vi "Set Scaling (MapRange).vi"(7 "Scaled Units":string, 8 "error in (no error)":errorcluster, 9 "Range":T1={"Minimum"=-5.0, "Maximum"=5.0}, 10 "Scale Name":string, 11 "DAQmx-AI":refnum<class "DAQmx-AI.lvclass">) -> (0 "error out":errorcluster, 3 "DAQmx-AI out":refnum<class "DAQmx-AI.lvclass">)   [LabVIEW 2016, in "DAQmx-AI.lvclass"]
uses:
  DAQmx-AI.lvclass
  Typedefs/Scaling(MapRange)--Cluster.ctl
  Typedefs/ScalingType--Enum.ctl
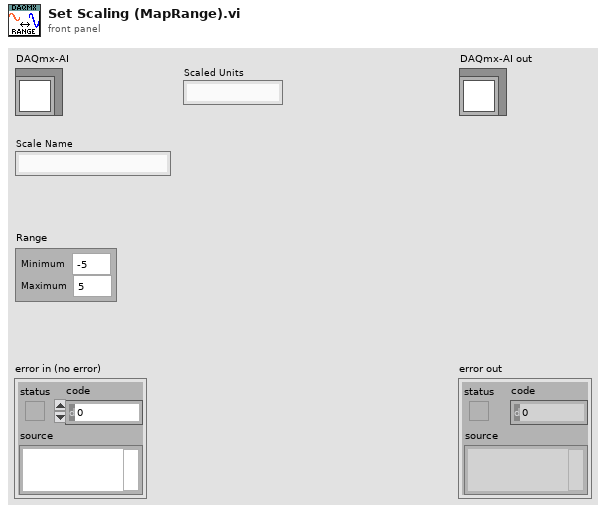
[diagram p1: front panel]
types:
  T1 = typedef "DAQmx-AI.lvclass/Scaling(MapRange)--Cluster.ctl" = cluster{"Minimum":dbl, "Maximum":dbl}
  T2 = typedef "DAQmx-AI.lvclass/ScalingType--Enum.ctl" = enum16{"No scaling", "Linear", "Map Range", "Polynomial", "Table"}
  T3 = typedef "DAQmx-AI.lvclass/Scaling--Cluster.ctl" = cluster{"Scale Name":string, "Scale Type":T2, "Scaled Units":string, "Linear":T4, "Map Range":T1, "Polynomial":T5, "Table":T6}
  T4 = typedef "DAQmx-AI.lvclass/Scaling(Linear)--Cluster.ctl" = cluster{"Slope":dbl, "Intercept":dbl}
  T5 = typedef "DAQmx-AI.lvclass/Scaling(Polynomial)--Cluster.ctl" = cluster{"forward coeff":dbl[], "reverse coeff":dbl[]}
  T6 = typedef "DAQmx-AI.lvclass/Scaling(Table)--Cluster.ctl" = cluster{"scaled values":dbl[], "pres-scaled values":dbl[]}
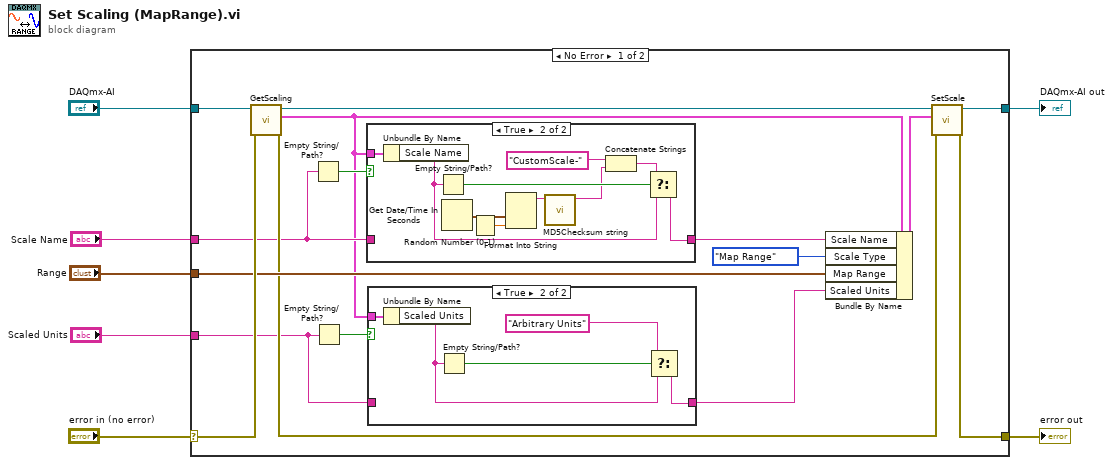
[diagram p0: block diagram]
diagram:
  n1 = case shown="No Error" "error in (no error)" {
    selector: "error in (no error)" -> [w19 w42]
    tunnel: [w22 w42] -> w6
    tunnel: [w23 w41] -> w4
    tunnel: "DAQmx-AI" -> [w21 w41]
    tunnel: "Scale Name" -> [w13 _]
    tunnel: "Scaled Units" -> [w8 _]
    tunnel: "Range" -> [w17 _]
    frame No Error {
      n2 = call "GetScaling.vi"("error in (no error)"=w19, "DAQmx-AI"=w21) -> ("error out"=w15:errorcluster, "Scaling"=w10:T3, "DAQmx-AI out"=w20:refnum<class "DAQmx-AI.lvclass">)  [unwired: 6 in, 1 out]
      n3 = Empty String/Path?(string/path=w13) -> (empty?=w14:bool)
      n4 = Empty String/Path?(string/path=w8) -> (empty?=w11:bool)
      n5 = case shown="True" w14 {
        tunnel: w10 -> [_ w40]
        tunnel: w13 -> [w30 _]
        tunnel: [w30 w37] -> w12
        frame False {
        }
        frame True {
          n6 = Unbundle By Name(w40) -> ("Scale Name"=w38:string)
          n7 = Empty String/Path?(string/path=w38) -> (empty?=w39:bool)
          n8 = Get Date/Time In Seconds() -> (seconds since 1Jan1904=w36:timestamp)
          n9 = Random Number (0-1)() -> (number: 0 to 1=w35:dbl)
          n10 = Format Into String(w36, w35) -> (resulting string=w34:string)  [unwired: 3 in, 1 out]
          n11 = call <vilib>:"MD5Checksum string.vi"("Message String"=w34) -> ("MD5 message-digest"=w32:string)  [unwired: 10 in]
          n12 = Concatenate Strings("CustomScale-" ("t"), w32) -> (w31:string)
          n13 = Select(t=w31, s=w39, f=w38) -> (s? t:f=w37:string)
        }
      }
      n14 = case shown="True" w11 {
        tunnel: w10 -> [_ w29]
        tunnel: w8 -> [w24 _]
        tunnel: [w24 w26] -> w9
        frame False {
        }
        frame True {
          n15 = Unbundle By Name(w29) -> ("Scaled Units"=w27:string)
          n16 = Empty String/Path?(string/path=w27) -> (empty?=w28:bool)
          n17 = Select(t="Arbitrary Units", s=w28, f=w27) -> (s? t:f=w26:string)
        }
      }
      n18 = Bundle By Name(cluster=w10, "Scale Name"=w12, "Scale Type"=ScalingType--Enum."Map Range", "Map Range"=w17, "Scaled Units"=w9) -> (w16:T3)
      n19 = call "SetScale.vi"("error in (no error)"=w15, "Scaling"=w16, "DAQmx-AI"=w20) -> ("error out"=w22:errorcluster, "DAQmx-AI out"=w23:refnum<class "DAQmx-AI.lvclass">)  [unwired: 7 in]
    }
    frame Error {
    }
  }
  "error out" <- w6
  "DAQmx-AI out" <- w4
